vi "LDA_meas_global_1.vi"() -> ()   [LabVIEW 2011]
uses:
  Controls/BSA_info_Cluster.ctl
  LDA/BSA_Type.ctl
panel:
  in  "Non-coincident":bool
  in  "Min Blue Shifted Power mW":i32
  in  "Min Blue Unshifted Power mW":i32
  in  "Min Green Shifted Power mW":i32
  in  "Min Green Unshifted Power mW":i32
  in  "LDA Results file Values":string[](array[string])
  in  "LDA Results file headers":string[](array[string])
  in  "Transit times":dbl[](array[numeric]) format="%.2f"
  in  "Additional BSA1 Setup":string
  in  "Max Record length BSA1":dbl=2.0 format="%.2f"
  in  "BSA Type":T1
  out "LDA Scale and Offset":T2(array[cluster])
  out "Max Vel BSA1":dbl=7.733999999999999 format="%.2f"
  out "Min Vel BSA1":dbl format="%.2f"
  out "High Volt BSA1":i16=2000 min=0 max=2040 step=8
  out "Signal gain BSA1":i16=30 min=0 max=57 step=1
  in  "BSA IP Number":string
  in  "Using 45 Degree Mirror?":bool
  in  "LDA Timescales":dbl[](array[numeric]) format="%.2f"
  in  "Buffer mode":enum16{"One shot", "Ring", "FIFO"}(ring)
  out "Optic Calib factor BSA1":dbl=3.867 format="%.4e"
  in  "Focal Length (mm)":dbl
  in  "Beam Separation (mm)":dbl
  in  "Probe Configuration":string
  in  "Multiply Velocity by -1":bool
  in  "Sync Delay Time (ms)":dbl=24.0 format="%.2f"
  in  "Time for last Block (s)":dbl=1000.0 format="%.2f"
  in  "ADC Frequency Hz":dbl=1000.0 format="%.2f"
  out "Vel Comp BSA1":string="U"
  in  "LDA stats type":string
  in  "Arrival times":dbl[](array[numeric]) format="%.2f"
  out "BSA1 info":T3={"GPIB Address"="13", "No of Check Bytes"=4, "Extra Info"="57N11", "COLOUR"=52224, "Wavelength (nm)"=52224.0} {"Wavelength (nm)" format="%.1f"}
  in  "data type":T4(array[ring])=[enum."Velocity", enum."Arrival time"]
  in  "Number of measured quantities":i32=2
  in  "Bandwidth BSA1":dbl=7.734 format="%.2f"
  in  "Centre Freq BSA1":dbl=3.867 format="%.2f"
  out "Anode current limit (mA)":T5(ring)=enum."0.1"
  in  "Record length BSA1":dbl=2.0 format="%.2f"
  out "Output":T6={"Output data format"=enum."Velocity, arrival time", "Non-validated signals"=enum."Accept"}
  out "Range":T7={"Centre frequency"=20, "Bandwidth"=11, "Units"=enum."m/s", "Frequency shift"=enum."Enabled"} {"Bandwidth" items=["3.877E-3", "7.754E-3", "15.508E-3", "31.016E-3", "62.031E-3", "124.063E-3", "248.125E-3", "496.250E-3", "992.500E-3", "1.985E+0", "3.970E+0", "7.940E+0", "15.880E+0", "31.760E+0"]; "Centre frequency" items=["-15.880E+0", "-14.888E+0", "-13.895E+0", "-12.902E+0", "-11.910E+0", "-10.918E+0", "-9.925E+0", "-8.933E+0", "-7.940E+0", "-6.947E+0", "-5.955E+0", "-4.963E+0", "-3.970E+0", "-2.978E+0", "-1.985E+0", "-992.500E-3", "0.000E+0", "992.500E-3", "1.985E+0", "2.978E+0", "3.970E+0", "4.963E+0", "5.955E+0", "6.947E+0", "7.940E+0", "8.933E+0", "9.925E+0", "10.918E+0", "11.910E+0", "12.902E+0", "13.895E+0", "14.888E+0", "15.880E+0"]}
  out "Analysis parameters":T8={"Burst criterion"=enum."Envelope", "Oversize reject level"=enum."1 (disabled)", "Pedestal attenuation"=enum."0", "Record length"=enum."32", "Quality factor"=0} {"Quality factor" min=0 max=80 step=10}
  out "Data collection mode":T9 {"Duty cycle (%)" format="%.2f"; "Dead time (s)" format="%.2f"}
  out "Clock parameters":T10={"Arrival time clock"=enum."Internal", "Clock source"=enum."Master", "Coincidence"=enum."Master"}
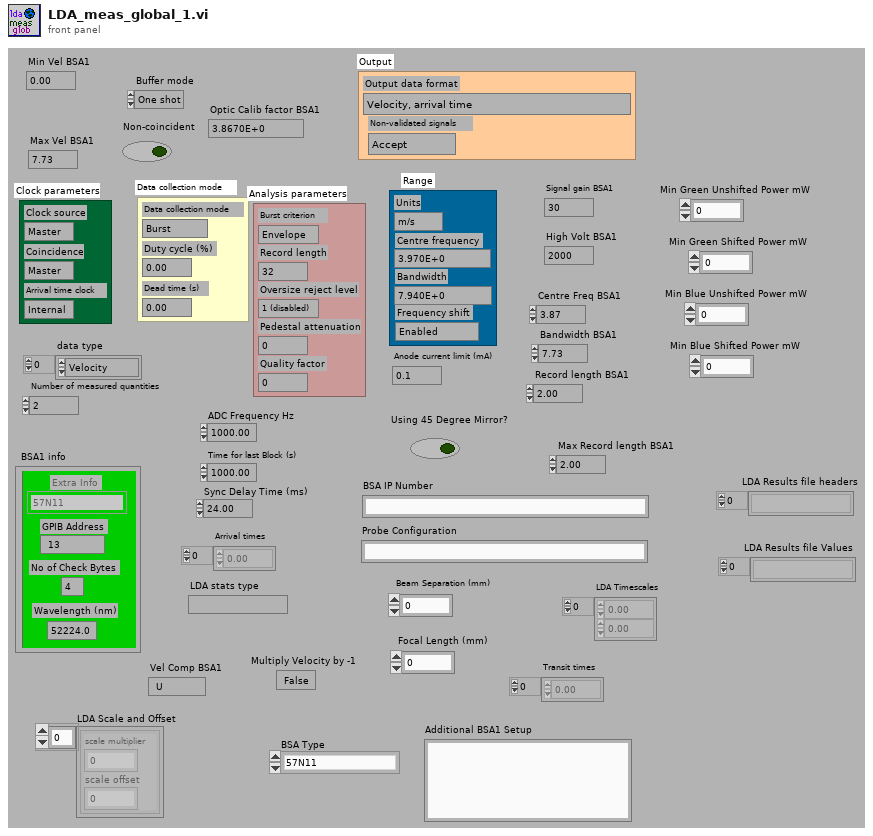
[diagram p1: front panel]
types:
  T1 = typedef "BSA_Type.ctl" = enum16{"57N11", "BSA F60"}
  T2 = cluster{"scale multiplier":dbl, "scale offset":dbl}[]
  T3 = typedef "BSA_info_Cluster.ctl" = cluster{"GPIB Address":string, "No of Check Bytes":i32, "Extra Info":string, "COLOUR":u32, "Wavelength (nm)":dbl}
  T4 = enum16{"Velocity", "Transit time", "Arrival time"}[]
  T5 = enum16{"6.4", "3.2", "1.6", "0.8", "0.4", "0.2", "0.1", "0.05"}
  T6 = cluster{"Output data format":enum16{"Velocity, transit time, arrival time", "Velocity, arrival time", "Velocity, transit time", "Velocity"}, "Non-validated signals":enum16{"Accept", "Reject"}}
  T7 = cluster{"Centre frequency":u16, "Bandwidth":u16, "Units":enum16{"Hz", "m/s"}, "Frequency shift":enum16{"Disabled", "Enabled"}}
  T8 = cluster{"Burst criterion":enum16{"Envelope", "Pedestal", "Env and ped"}, "Oversize reject level":enum16{"1 (disabled)", "2", "3", "4", "5", "6", "7", "8", "9"}, "Pedestal attenuation":enum16{"0", "6", "12", "18"}, "Record length":enum16{"8", "16", "32", "64"}, "Quality factor":i16}
  T9 = cluster{"Dead time (s)":dbl, "Duty cycle (%)":dbl, "Data collection mode":enum16{"Burst", "Contiuous", "Dead time", "External"}}
  T10 = cluster{"Arrival time clock":enum16{"External", "Internal"}, "Clock source":enum16{"Slave", "Master", "Private"}, "Coincidence":enum16{"Slave", "Master", "Private"}}
diagram:
